vi "Add Items to Targets.vi"(8 "error in (no error)":errorcluster, 9 "Items in":T1[](array[typedef]), 10 "Target Names in":string[](array[string]), 11 "Project Sync Tools in":refnum<class "Project Sync Tools.lvclass">) -> (0 "error out":errorcluster, 1 "Items out":T1[](array[typedef]), 2 "Target Names out":string[](array[string]), 3 "Project Sync Tools out":refnum<class "Project Sync Tools.lvclass">)   [LabVIEW 2019, in "Project Sync Tools.lvclass"]
uses:
  Project Sync Tools.lvclass
  TypeDefs/Item Settings.ctl
  Project Sync Tools.lvclass/Project Sync Tools.ctl
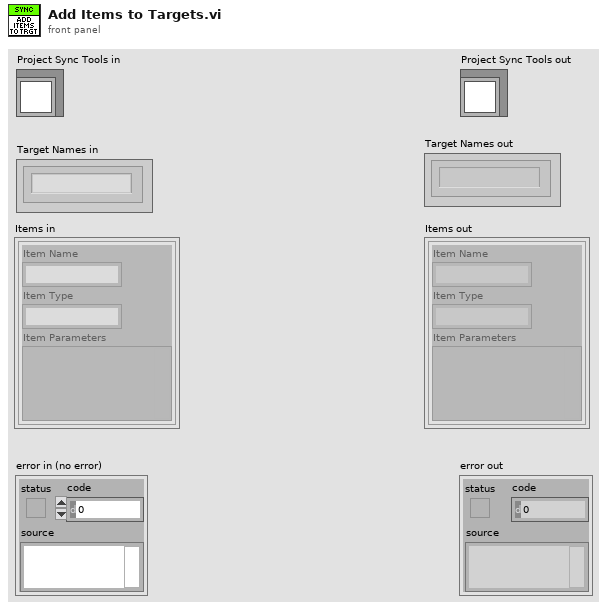
[diagram p1: front panel]
types:
  T1 = typedef "Project Sync Tools.lvclass/Item Settings.ctl" = cluster{"Item Name":string, "Item Type":string, "Item Parameters":variant}
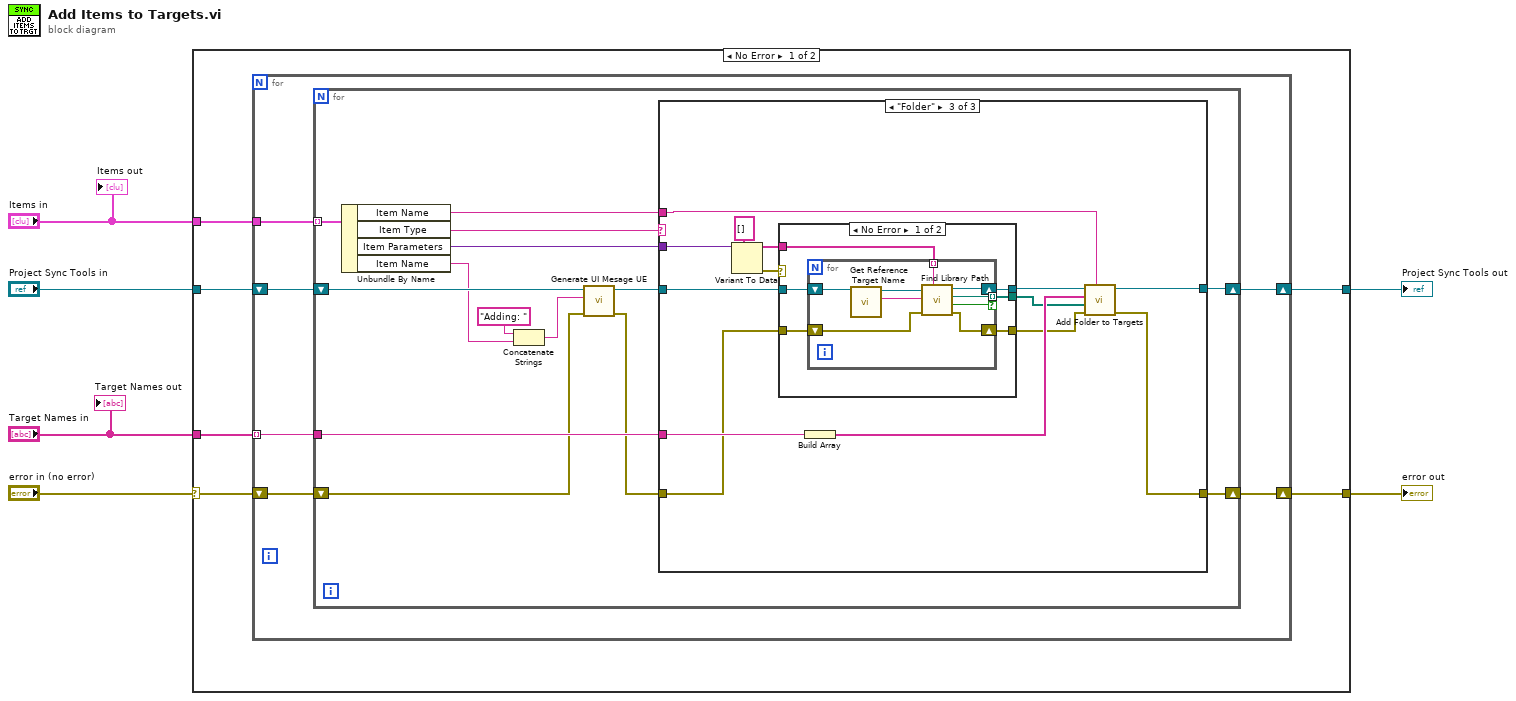
[diagram p0: block diagram]
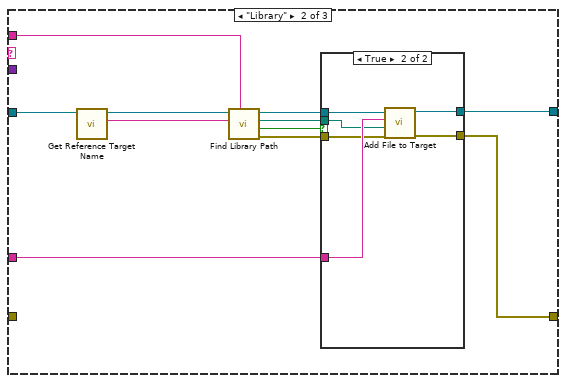
[diagram p3: hidden frame]
diagram:
  n1 = case shown="No Error" "error in (no error)" {
    selector: "error in (no error)" -> [w8 w86]
    tunnel: [w7 w86] -> w5
    tunnel: [w9 w85] -> w3
    tunnel: "Project Sync Tools in" -> [w10 w85]
    tunnel: "Target Names in" -> [w12 _]
    tunnel: "Items in" -> [w11 _]
    frame No Error {
      n2 = for {
        tunnel: w12 -> [w16] mode=indexing
        tunnel: w11 -> [w18]
        shift-right: [w15] -> w9
        shift-left: w10 -> [w17]
        shift-right: [w13] -> w7
        shift-left: w8 -> [w14]
        n3 = for {
          tunnel: w18 -> [w32] mode=indexing
          shift-right: [w28] -> w15
          shift-left: w17 -> [w25]
          tunnel: w16 -> [w29]
          shift-right: [w26] -> w13
          shift-left: w14 -> [w24]
          n4 = Unbundle By Name(w32) -> ("Item Name"=w30:string, "Item Type"=w31:string, "Item Parameters"=w27:variant, "Item Name"=w20:string)
          n5 = Concatenate Strings("Adding: " ("UI Message"), w20) -> (w19:string)
          n6 = call "Generate UI Mesage UE.vi"("error in (no error)"=w24, "UI Message"=w19, "Project Sync Tools in"=w25) -> ("error out"=w22:errorcluster, "Project Sync Tools out"=w23:refnum<class "Project Sync Tools.lvclass">)  [unwired: 7 in]
          n7 = case shown="\"Folder\"" w31 {
            tunnel: w23 -> [w34 w44 w65]
            tunnel: w30 -> [_ w45 w61]
            tunnel: w29 -> [_ w40 w60]
            tunnel: [w34 w38 w56] -> w28
            tunnel: w27 -> [_ _ w67]
            tunnel: [w33 w35 w55] -> w26
            tunnel: w22 -> [w33 _ w54]
            frame "None", Default {
            }
            frame "Library" {
              n8 = call "Get Reference Target Name.vi"("Project Sync Tools in"=w44) -> ("Reference Target Name"=w42:string, "Project Sync Tools out"=w43:refnum<class "Project Sync Tools.lvclass">)  [unwired: 9 in]
              n9 = call "Find Library Path.vi"("Library Name"=w45, "Target Name"=w42, "Project Sync Tools in"=w43) -> ("error out"=w37:errorcluster, "Found"=w36:bool, "Library Path"=w39:path, "Project Sync Tools out"=w41:refnum<class "Project Sync Tools.lvclass">)  [unwired: 5 in]
              n10 = case shown="True" w36 {
                tunnel: w41 -> [w47 w53]
                tunnel: w40 -> [_ w52]
                tunnel: w39 -> [_ w51]
                tunnel: [w47 w50] -> w38
                tunnel: w37 -> [w46 w49]
                tunnel: [w46 w48] -> w35
                frame False {
                }
                frame True {
                  n11 = call "Add File to Target.vi"("error in (no error)"=w49, "Flie Path"=w51, "Target Name"=w52, "Project Sync Tools in"=w53) -> ("error out"=w48:errorcluster, "Project Sync Tools out"=w50:refnum<class "Project Sync Tools.lvclass">)  [unwired: 6 in]
                }
              }
            }
            frame "Folder" {
              n12 = Variant To Data(type=string[] [] ("Filtered Names"), Variant=w67) -> (data=w63:string[], error out=w64:errorcluster)  [unwired: 1 in]
              n13 = case shown="No Error" w64 {
                tunnel: w65 -> [w73 w83]
                tunnel: w54 -> [w72 w84]
                tunnel: w63 -> [w71 _]
                tunnel: [w70 w84] -> w57
                tunnel: [w69 w83] -> w62
                tunnel: [w68 _] -> w58
                frame No Error {
                  n14 = for {
                    tunnel: w71 -> [w78] mode=indexing
                    tunnel: [w77] -> w68 mode=indexing if=w76
                    shift-right: [w75] -> w69
                    shift-left: w73 -> [w82]
                    shift-right: [w74] -> w70
                    shift-left: w72 -> [w79]
                    n15 = call "Get Reference Target Name.vi"("Project Sync Tools in"=w82) -> ("Reference Target Name"=w80:string, "Project Sync Tools out"=w81:refnum<class "Project Sync Tools.lvclass">)  [unwired: 9 in]
                    n16 = call "Find Library Path.vi"("Library Name"=w78, "error in (no error)"=w79, "Target Name"=w80, "Project Sync Tools in"=w81) -> ("error out"=w74:errorcluster, "Found"=w76:bool, "Library Path"=w77:path, "Project Sync Tools out"=w75:refnum<class "Project Sync Tools.lvclass">)  [unwired: 4 in]
                  }
                }
                frame Error {
                }
              }
              n17 = Build Array(w60) -> (w59:string[])
              n18 = call "Add Folder to Targets.vi"("Folder Name"=w61, "error in (no error)"=w57, "Content Paths"=w58, "Target Names"=w59, "Project Sync Tools in"=w62) -> ("error out"=w55:errorcluster, "Project Sync Tools out"=w56:refnum<class "Project Sync Tools.lvclass">)  [unwired: 5 in]
            }
          }
        }
      }
    }
    frame Error {
    }
  }
  "error out" <- w5
  "Project Sync Tools out" <- w3
  "Items out" <- "Items in"
  "Target Names out" <- "Target Names in"
